vi "Assignment6_CarGate.vi"   [LabVIEW 2024]
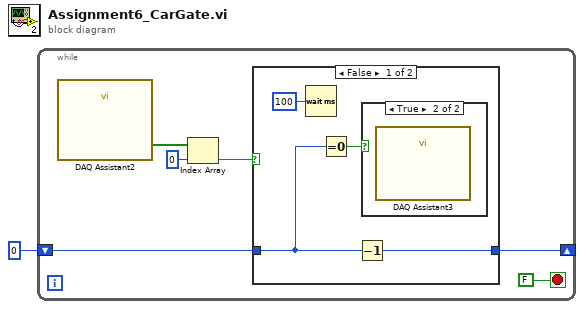
[diagram p0: block diagram]
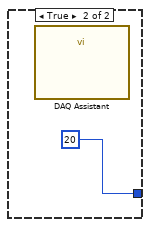
[diagram p3: hidden frame]
diagram:
  n1 = while {
    shift-right: [w4] -> _
    shift-left: 0 -> [w3]
    stop <- FALSE stop-if-true
    n2 = call "DAQ Assistant2"() -> ("data"=w5:bool[])  [unwired: 17 in, 2 out]
    n3 = Index Array(array=w5, index=0) -> (element=w2:bool)
    n4 = case shown="False" w2 {
      tunnel: [w10 20] -> w4
      tunnel: w3 -> [w9 _]
      frame False {
        n5 = Wait (ms)(milliseconds to wait=u32 100) -> ()  [unwired: 1 out]
        n6 = Equal To 0?(x=w9) -> (x = 0?=w8:bool)
        n7 = Decrement(x=w9) -> (x-1=w10:i32)
        n8 = case shown="True" w8 {
          frame False {
          }
          frame True {
            n9 = call "DAQ Assistant3"() -> ()  [unwired: 18 in, 2 out]
          }
        }
      }
      frame True {
        n10 = call "DAQ Assistant"() -> ()  [unwired: 18 in, 2 out]
      }
    }
  }
